vi "BME280-FormulaNode_Compensation.vi"   [LabVIEW 2015]
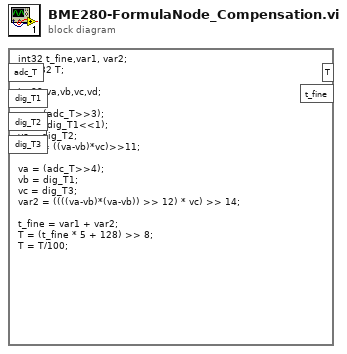
[diagram p0: block diagram]
diagram:
  n1 = formula code="int32 t_fine,var1, var2; \nfloat32 T;\n\nint32 va,vb,vc,vd;\n\nva = (adc_T>>3);\nvb = (dig_T1<<1);\nvc = dig_T2;\nvar1 = ((va-vb)*vc)>>11;\n\nva = (adc_T>>4);\nvb = dig_T1;\nvc = dig_T3;\nvar2 = ((((va-vb)*(va-vb)) >> 12) * vc) >> 14;\n\nt_fine = var1 + var2;\nT = (t_fine * 5 + 128) >> 8;\nT = T/100;"() -> ()  [unwired: 4 in, 2 out]
